vi "rszvl_core_global.vi"() -> ()   [LabVIEW 2014] (continued)
a stopped measurement at the current position in single sweep mode. The function is useful especially for trace functions MAXHold, MINHold and AVERage if the previous results are not to be cleared with Sweep Count > 0 or Average Count > 0 on restarting the measurement (INIT:IMMediate resets the previous results on restarting the measurement).\nThe single-sweep mode is automatically switched on. Synchronization to the end of the indicated number of measurements can then be performed with the command *OPC, *OPC? or *WAI. In the continuous-sweep mode, synchronization to the sweep end is not possible since the overall measurement never ends.", "Flags"={"OPC Wait"=FALSE, "Dont check status"=FALSE, "*WAI"=FALSE}, "Check Status Callback"=""}, {"Level"=3, "Descriptive Name"="Abort", "Class Only"=FALSE, "Data Type"=4, "Access"=1, "Identifier"="RSZVL_ATTR_MEAS_ABORT", "Range Table"="", "Command"="ABOR", "Read Callback"="", "Write Callback"="", "Range Callback"="", "Check Callback"="", "Rngtable Callback"="", "Coerce Callback"="", "User Callback"="", "Supported Models"="", "Instrument Options"="", "Repeated Capabilities"="", "Restricted Repeated Capabilities"="", "Help"="This attribute aborts a current measurement and resets the trigger system.\n\nAvailable Repeated Capabilities:\nNone\n\nRemote-control command(s):\nABORt", "Flags"={"OPC Wait"=FALSE, "Dont check status"=FALSE, "*WAI"=FALSE}, "Check Status Callback"=""}, {"Level"=3, "Descriptive Name"="Initiate", "Class Only"=FALSE, "Data Type"=4, "Access"=1, "Identifier"="RSZVL_ATTR_INIT", "Range Table"="", "Command"="INIT;*WAI", "Read Callback"="", "Write Callback"="", "Range Callback"="", "Check Callback"="", "Rngtable Callback"="", "Coerce Callback"="", "User Callback"="", "Supported Models"="", "Instrument Options"="", "Repeated Capabilities"="", "Restricted Repeated Capabilities"="", "Help"="This attribute initiates a new sweep.\nIn single sweep mode, synchronization to the end of the indicated number of measurements is achieved with the command *OPC. In continuous-sweep mode, synchronization to the sweep end is not possible since the overall measurement never ends.\n\nAvailable Repeated Capabilities:\nNone\n\nRemote-control command(s):\nINITiate[:IMMediate]", "Flags"={"OPC Wait"=TRUE, "Dont check status"=FALSE, "*WAI"=FALSE}, "Check Status Callback"=""}, {"Level"=3, "Descriptive Name"="Initiate Continuous", "Class Only"=FALSE, "Data Type"=3, "Access"=2, "Identifier"="RSZVL_ATTR_INIT_CONT", "Range Table"="", "Command"="INIT:CONT", "Read Callback"="", "Write Callback"="", "Range Callback"="", "Check Callback"="", "Rngtable Callback"="", "Coerce Callback"="", "User Callback"="", "Supported Models"="", "Instrument Options"="", "Repeated Capabilities"="", "Restricted Repeated Capabilities"="", "Help"="This attribute determines whether the trigger system is continuously initiated (continuous) or performs single measurements (single).\nIn the spectrum analysis mode, this setting refers to the sweep sequence (switching between continuous/single sweep).\n\nAvailable Repeated Capabilities:\nNone\n\nRemote-control command(s):\nINITiate<1|2>:CONTinuous ON | OFF", "Flags"={"OPC Wait"=FALSE, "Dont check status"=FALSE, "*WAI"=FALSE}, "Check Status Callback"=""}, {"Level"=3, "Descriptive Name"="Send Software Trigger", "Class Only"=FALSE, "Data Type"=4, "Access"=1, "Identifier"="RSZVL_ATTR_INIT_SW_TRIGGER", "Range Table"="", "Command"="*TRG", "Read Callback"="", "Write Callback"="", "Range Callback"="", "Check Callback"="", "Rngtable Callback"="", "Coerce Callback"="", "User Callback"="", "Supported Models"="", "Instrument Options"="", "Repeated Capabilities"="", "Restricted Repeated Capabilities"="", "Help"="This attribute sends a software trigger to the instrument.\n\nAvailable Repeated Capabilities:\nNone\n\nRemote-control command(s):\n*TRG", "Flags"={"OPC Wait"=TRUE, "Dont check status"=FALSE, "*WAI"=FALSE}, "Check Status Callback"=""}, {"Level"=3, "Descriptive Name"="Continue Measurement", "Class Only"=FALSE, "Data Type"=4, "Access"=1, "Identifier"="RSZVL_ATTR_INIT_CONMEAS", "Range Table"="", "Command"="INIT:CONM;*WAI", "Read Callback"="", "Write Callback"="", "Range Callback"="", "Check Callback"="", "Rngtable Callback"="", "Coerce Callback"="", "User Callback"="", "Supported Models"="", "Instrument Options"="", "Repeated Capabilities"="", "Restricted Repeated Capabilities"="", "Help"="This attribute continues a stopped measurement at the current position in single sweep mode. The function is useful especially for trace functions MAXHold, MINHold and AVERage if the previous results are not to be cleared with Sweep Count > 0 or Average Count > 0 on restarting the measurement (INIT:IMMediate resets the previous results on restarting the measurement).\nThe single-sweep mode is automatically switched on. Synchronization to the end of the indicated number of measurements can then be performed with the command *OPC, *OPC? or *WAI. In the continuous-sweep mode, synchronization to the sweep end is not possible since the overall measurement never ends.\n\nAvailable Repeated Capabilities:\nNone\n\nRemote-control command(s):\nINITiate<1|2>:CONMeas", "Flags"={"OPC Wait"=TRUE, "Dont check status"=FALSE, "*WAI"=FALSE}, "Check Status Callback"=""}, {"Level"=2, "Descriptive Name"="Average", "Class Only"=TRUE, "Data Type"=0, "Access"=0, "Identifier"="", "Range Table"="", "Command"="", "Read Callback"="", "Write Callback"="", "Range Callback"="", "Check Callback"="", "Rngtable Callback"="", "Coerce Callback"="", "User Callback"="", "Supported Models"="", "Instrument Options"="", "Repeated Capabilities"="", "Restricted Repeated Capabilities"="", "Help"="This subsystem calculates the average of the acquired data.\n\n(1) Averaging State:\nThis attribute switches on or off the average calculation for the selected trace.\n\n(2) Averaging Type:\nThis attribute selects the type of average function. If Video is selected, the logarithmic power is averaged and, if Linear is selected, the power values are averaged before they are converted to logarithmic values. The type of average calculation is equally set for all traces\n\n(3) Averaging Count:\nThis attribute defines the number of measurements which contribute to the average value.\nIt should be noted that continuous averaging will be performed after the indicated number has been reached in continuous sweep mode.\nIn single sweep mode, the sweep is stopped as soon as the indicated number of measurements (sweeps) is reached. Synchronization to the end of the indicated number of measurements is only possible in single sweep mode.\n\n(4) Averaging Count Auto:\nThis attribute is implemented only for reasons of compatibility with the FSP family. It selects a suitable number of counts for the selected measurement type.", "Flags"={"OPC Wait"=FALSE, "Dont check status"=FALSE, "*WAI"=FALSE}, "Check Status Callback"=""}, {"Level"=3, "Descriptive Name"="Averaging State", "Class Only"=FALSE, "Data Type"=3, "Access"=2, "Identifier"="RSZVL_ATTR_AVG_STATE", "Range Table"="", "Command"="SENS:AVER:STAT{Trace}", "Read Callback"="", "Write Callback"="", "Range Callback"="", "Check Callback"="", "Rngtable Callback"="", "Coerce Callback"="", "User Callback"="", "Supported Models"="", "Instrument Options"="", "Repeated Capabilities"="", "Restricted Repeated Capabilities"="", "Help"="This attribute switches on or off the average calculation for the selected trace.\n\nAvailable Repeated Capabilities:\nTrace: TR1,TR2,TR3,TR4,TR5,TR6,TR7,TR8,TR9,TR10,TR11,TR12,TR13,TR14,TR15,TR16,TR17,TR18,TR19,TR20\r\n\nRemote-control command(s):\n[SENSe<1|2>:]AVERage[:STATe<1 to 3>] ON | OFF", "Flags"={"OPC Wait"=FALSE, "Dont check status"=FALSE, "*WAI"=FALSE}, "Check Status Callback"=""}, {"Level"=3, "Descriptive Name"="Averaging Type", "Class Only"=FALSE, "Data Type"=0, "Access"=2, "Identifier"="RSZVL_ATTR_AVG_TYPE", "Range Table"="rszvl_rngAvgType", "Command"="SENS:AVER:TYPE", "Read Callback"="", "Write Callback"="", "Range Callback"="", "Check Callback"="", "Rngtable Callback"="", "Coerce Callback"="", "User Callback"="", "Supported Models"="", "Instrument Options"="", "Repeated Capabilities"="", "Restricted Repeated Capabilities"="", "Help"="This attribute selects the type of average function. If Video is selected, the logarithmic power is averaged and, if Linear is selected, the power values are averaged before they are converted to logarithmic values. The type of average calculation is equally set for all traces\n\nAvailable Repeated Capabilities:\nNone\n\nRemote-control command(s):\n[SENSe<1|2>:]AVERage:TYPE VIDeo | LINear", "Flags"={"OPC Wait"=FALSE, "Dont check status"=FALSE, "*WAI"=FALSE}, "Check Status Callback"=""}, {"Level"=3, "Descriptive Name"="Averaging Count", "Class Only"=FALSE, "Data Type"=0, "Access"=2, "Identifier"="RSZVL_ATTR_AVG_COUNT", "Range Table"="rszvl_rngAvgCount", "Command"="SENS:AVER:COUN", "Read Callback"="", "Write Callback"="", "Range Callback"="", "Check Callback"="", "Rngtable Callback"="", "Coerce Callback"="", "User Callback"="", "Supported Models"="", "Instrument Options"="", "Repeated Capabilities"="", "Restricted Repeated Capabilities"="", "Help"="This attribute defines the number of measurements which contribute to the average value.\nIt should be noted that continuous averaging will be performed after the indicated number has been reached in continuous sweep mode.\nIn single sweep mode, the sweep is stopped as soon as the indicated number of measurements (sweeps) is reached. Synchronization to the end of the indicated number of measurements is only possible in single sweep mode.\n\nAvailable Repeated Capabilities:\nNone\n\nRemote-control command(s):\n[SENSe<1|2>:]AVERage:COUNt", "Flags"={"OPC Wait"=FALSE, "Dont check status"=FALSE, "*WAI"=FALSE}, "Check Status Callback"=""}, {"Level"=3, "Descriptive Name"="Averaging Count Auto", "Class Only"=FALSE, "Data Type"=3, "Access"=2, "Identifier"="RSZVL_ATTR_AVG_COUNT_AUTO", "Range Table"="", "Command"="SENS:AVER:COUN:AUTO", "Read Callback"="", "Write Callback"="", "Range Callback"="", "Check Callback"="", "Rngtable Callback"="", "Coerce Callback"="", "User Callback"="", "Supported Models"="", "Instrument Options"="", "Repeated Capabilities"="", "Restricted Repeated Capabilities"="", "Help"="This attribute is implemented only for reasons of compatibility with the FSP family. It selects a suitable number of counts for the selected measurement type.\n\nAvailable Repeated Capabilities:\nNone\n\nRemote-control command(s):\n[SENSe<1|2>:]AVERage:COUNt:AUTO", "Flags"={"OPC Wait"=FALSE, "Dont check status"=FALSE, "*WAI"=FALSE}, "Check Status Callback"=""}, {"Level"=2, "Descriptive Name"="Bandwidth", "Class Only"=TRUE, "Data Type"=0, "Access"=0, "Identifier"="", "Range Table"="", "Command"="", "Read Callback"="", "Write Callback"="", "Range Callback"="", "Check Callback"="", "Rngtable Callback"="", "Coerce Callback"="", "User Callback"="", "Supported Models"="", "Instrument Options"="", "Repeated Capabilities"="", "Restricted Repeated Capabilities"="", "Help"="This class contains attributes configuring resolution and video bandwidth.\n\n(1) Resolution Bandwidth Filter Type:\nThis attribute sets the filter type for the resolution bandwidth.\n\n(2) Video Bandwidth Filter Type:\nThis attribute selects the position of the video filter in the signal path, provided that the resolution bandwidth is <=100 kHz:", "Flags"={"OPC Wait"=FALSE, "Dont check status"=FALSE, "*WAI"=FALSE}, "Check Status Callback"=""}, {"Level"=3, "Descriptive Name"="Resolution Bandwidth Filter Type", "Class Only"=FALSE, "Data Type"=0, "Access"=2, "Identifier"="RSZVL_ATTR_RESOLUTION_BANDWIDTH_FILTER_TYPE", "Range Table"="rszvl_rngBandFiltType", "Command"="SENS:BAND:TYPE", "Read Callback"="", "Write Callback"="", "Range Callback"="", "Check Callback"="", "Rngtable Callback"="", "Coerce Callback"="", "User Callback"="", "Supported Models"="", "Instrument Options"="", "Repeated Capabilities"="", "Restricted Repeated Capabilities"="", "Help"="This attribute sets the filter type for the resolution bandwidth.\n\nThe possible combinations of filter type and filter bandwidth are listed in Operating Manual in the table List of available channel filters in chapter 4, section Setting Bandwidths and Sweep Time- Key BW.\n\nAvailable Repeated Capabilities:\nNone\n\nRemote-control command(s):\n[SENSe<1|2>:]BANDwidth|BWIDth[:RESolution]:TYPE NORMal | FFT | CFILter | RRC | PULSe", "Flags"={"OPC Wait"=FALSE, "Dont check status"=FALSE, "*WAI"=FALSE}, "Check Status Callback"=""}, {"Level"=3, "Descriptive Name"="Video Bandwidth Filter Type", "Class Only"=FALSE, "Data Type"=0, "Access"=2, "Identifier"="RSZVL_ATTR_VIDEO_BANDWIDTH_TYPE", "Range Table"="rszvl_rngLinLog", "Command"="SENS:BAND:VID:TYPE", "Read Callback"="", "Write Callback"="", "Range Callback"="", "Check Callback"="", "Rngtable Callback"="", "Coerce Callback"="", "User Callback"="", "Supported Models"="", "Instrument Options"="", "Repeated Capabilities"="", "Restricted Repeated Capabilities"="", "Help"="This attribute selects the position of the video filter in the signal path, provided that the resolution bandwidth is <=100 kHz:\n\nAvailable Repeated Capabilities:\nNone\n\nRemote-control command(s):\n[SENSe<1|2>:]BANDwidth|BWIDth:VIDeo:TYPE LINear | LOGarithmic", "Flags"={"OPC Wait"=FALSE, "Dont check status"=FALSE, "*WAI"=FALSE}, "Check Status Callback"=""}, {"Level"=2, "Descriptive Name"="Trace", "Class Only"=TRUE, "Data Type"=0, "Access"=0, "Identifier"="", "Range Table"="", "Command"="", "Read Callback"="", "Write Callback"="", "Range Callback"="", "Check Callback"="", "Rngtable Callback"="", "Coerce Callback"="", "User Callback"="", "Supported Models"="", "Instrument Options"="", "Repeated Capabilities"="", "Restricted Repeated Capabilities"="", "Help"="Trace settings and configuration.\n\n(1) Trace State:\nThis attribute switches on or off the display of the corresponding trace.\n\n(2) Trace Reset Behavior:\nThis attribute specifies whether or not the traces with peak or minimum value detection are reset after specific parameter changes.\n\n(3) Trace Type:\nThis attribute defines the type of display and the evaluation of the traces. WRITE corresponds to the Clr/Write mode of manual operation. The trace is switched off (= BLANK in manual operation) with DISP:WIND:TRAC:STAT OFF.\n\n(4) Trace Math State:\nThis attribute switches the mathematical relation of traces on or off.\n\n(5) Trace Math Position:\nThis attribute defines the position of the result of the trace mathematics. The indication is in % of the screen height, with 100% corresponding to the upper diagram border.\n\n(6) Detector Type:\nSpecifies the detection method used to capture and process the signal. This governs the data acquisition for a particular sweep, but does not have any control over how multiple sweeps are processed.\n\n(7) Detector Type Auto:\nEnables the auto detector.", "Flags"={"OPC Wait"=FALSE, "Dont check status"=FALSE, "*WAI"=FALSE}, "Check Status Callback"=""}, {"Level"=3, "Descriptive Name"="Trace State", "Class Only"=FALSE, "Data Type"=3, "Access"=2, "Identifier"="RSZVL_ATTR_TRACE_STATE", "Range Table"="", "Command"="DISP:WIND:TRACE{Trace}", "Read Callback"="", "Write Callback"="", "Range Callback"="", "Check Callback"="", "Rngtable Callback"="", "Coerce Callback"="", "User Callback"="", "Supported Models"="", "Instrument Options"="", "Repeated Capabilities"="", "Restricted Repeated Capabilities"="", "Help"="This attribute switches on or off the display of the corresponding trace.\n\nAvailable Repeated Capabilities:\nTrace: TR1,TR2,TR3,TR4,TR5,TR6,TR7,TR8,TR9,TR10,TR11,TR12,TR13,TR14,TR15,TR16,TR17,TR18,TR19,TR20\r\n\nRemote-control command(s):\nDISPlay[:WINDow<1|2>]:TRACE<1 to 6>[:STATe]", "Flags"={"OPC Wait"=FALSE, "Dont check status"=FALSE, "*WAI"=FALSE}, "Check Status Callback"=""}, {"Level"=3, "Descriptive Name"="Trace Reset Behavior", "Class Only"=FALSE, "Data Type"=3, "Access"=2, "Identifier"="RSZVL_ATTR_TRACE_RESET_BEHAVIOR", "Range Table"="", "Command"="DISP:WIND:TRAC{Trace}:MODE:HCON", "Read Callback"="", "Write Callback"="", "Range Callback"="", "Check Callback"="", "Rngtable Callback"="", "Coerce Callback"="", "User Callback"="", "Supported Models"="", "Instrument Options"="", "Repeated Capabilities"="", "Restricted Repeated Capabilities"="", "Help"="This attribute specifies whether or not the traces with peak or minimum value detection are reset after specific parameter changes.\nUsually the measurement must be restarted after a parameter change, before an evaluation of the measurement results is performed (e.g. with a marker). In cases in which a change causes a compulsory new measurement, the trace is automatically reset in order to prevent erroneous measurements of previous measurement results (e.g. when the span changes). For applications in which this behavior is not desired, this mechanism can be switched off.\n\nAvailable Repeated Capabilities:\nTrace: TR1,TR2,TR3,TR4,TR5,TR6,TR7,TR8,TR9,TR10,TR11,TR12,TR13,TR14,TR15,TR16,TR17,TR18,TR19,TR20\r\n\nRemote-control command(s):\nDISPlay[:WINDow<1|2>]:TRACe<1 to 6>:MODE:HCONtinuous ON | OFF", "Flags"={"OPC Wait"=FALSE, "Dont check status"=FALSE, "*WAI"=FALSE}, "Check Status Callback"=""}, {"Level"=3, "Descriptive Name"="Trace Type", "Class Only"=FALSE, "Data Type"=0, "Access"=2, "Identifier"="RSZVL_ATTR_TRACE_TYPE", "Range Table"="rszvl_rngTraceMode", "Command"="DISP:WIND:TRAC{Trace}:MODe", "Read Callback"="", "Write Callback"="", "Range Callback"="", "Check Callback"="", "Rngtable Callback"="", "Coerce Callback"="", "User Callback"="", "Supported Models"="", "Instrument Options"="", "Repeated Capabilities"="", "Restricted Repeated Capabilities"="", "Help"="This attribute defines the type of display and the evaluation of the traces. WRITE corresponds to the Clr/Write mode of manual operation. The trace is switched off (= BLANK in manual operation) with DISP:WIND:TRAC:STAT OFF.\nThe number of measurements for AVERage, MAXHold and MINHold is defined with the command SENSe:AVERage:COUNt or SENSe:SWEep:COUNt. It should be noted that synchronization to the end of the indicated number of measurements is only possible in single sweep mode. If calculation of average values is active, selection between logarithmic and linear averaging is possible. For more detail see command SENSe:AVERage:TYPE.\n\nAvailable Repeated Capabilities:\nTrace: TR1,TR2,TR3,TR4,TR5,TR6,TR7,TR8,TR9,TR10,TR11,TR12,TR13,TR14,TR15,TR16,TR17,TR18,TR19,TR20\r\n\nRemote-control command(s):\nDISPlay[:WINDow<1|2>]:TRACe<1 to 6>:MODE WRITe | VIEW | AVERage | MAXHold | MINHold | BLANk", "Flags"={"OPC Wait"=FALSE, "Dont check status"=FALSE, "*WAI"=FALSE}, "Check Status Callback"=""}, {"Level"=3, "Descriptive Name"="Trace Math State", "Class Only"=FALSE, "Data Type"=3, "Access"=2, "Identifier"="RSZVL_ATTR_TRACE_MATH_STATE", "Range Table"="", "Command"="CALC:MATH:STAT", "Read Callback"="", "Write Callback"="", "Range Callback"="", "Check Callback"="", "Rngtable Callback"="", "Coerce Callback"="", "User Callback"="", "Supported Models"="", "Instrument Options"="", "Repeated Capabilities"="", "Restricted Repeated Capabilities"="", "Help"="This attribute switches the mathematical relation of traces on or off.\n\nAvailable Repeated Capabilities:\nNone\n\nRemote-control command(s):\nCALCulate<1|2>:MATH:STATe ON | OFF", "Flags"={"OPC Wait"=FALSE, "Dont check status"=FALSE, "*WAI"=FALSE}, "Check Status Callback"=""}, {"Level"=3, "Descriptive Name"="Trace Math Position", "Class Only"=FALSE, "Data Type"=1, "Access"=2, "Identifier"="RSZVL_ATTR_TRACE_MATH_POSITION", "Range Table"="rszvl_rngTraceMathPosition", "Command"="CALC:MATH:POS", "Read Callback"="", "Write Callback"="", "Range Callback"="", "Check Callback"="", "Rngtable Callback"="", "Coerce Callback"="", "User Callback"="", "Supported Models"="", "Instrument Options"="", "Repeated Capabilities"="", "Restricted Repeated Capabilities"="", "Help"="This attribute defines the position of the result of the trace mathematics. The indication is in % of the screen height, with 100% corresponding to the upper diagram border.\n\nAvailable Repeated Capabilities:\nNone\n\nRemote-control command(s):\nCALCulate<1|2>:MATH:POSition", "Flags"={"OPC Wait"=FALSE, "Dont check status"=FALSE, "*WAI"=FALSE}, "Check Status Callback"=""}, {"Level"=3, "Descriptive Name"="Detector Type", "Class Only"=FALSE, "Data Type"=0, "Access"=2, "Identifier"="RSZVL_ATTR_DETECTOR_TYPE", "Range Table"="rszvl_rngDetectorTypeRangeTable", "Command"="SENS:DET{Trace}:FUNC", "Read Callback"="", "Write Callback"="", "Range Callback"="", "Check Callback"="", "Rngtable Callback"="", "Coerce Callback"="", "User Callback"="", "Supported Models"="", "Instrument Options"="", "Repeated Capabilities"="", "Restricted Repeated Capabilities"="", "Help"="Specifies the detection method used to capture and process the signal. This governs the data acquisition for a particular sweep, but does not have any control over how multiple sweeps are processed.\n\nAvailable Repeated Capabilities:\nTrace: TR1,TR2,TR3,TR4,TR5,TR6,TR7,TR8,TR9,TR10,TR11,TR12,TR13,TR14,TR15,TR16,TR17,TR18,TR19,TR20\r\n\nRemote-control command(s):\n[SENSe<1|2>:]DETector<1 to 6>[:FUNCtion] APEak | NEGative | POSitive | SAMPle | RMS |", "Flags"={"OPC Wait"=FALSE, "Dont check status"=FALSE, "*WAI"=FALSE}, "Check Status Callback"=""}, {"Level"=3, "Descriptive Name"="Detector Type Auto", "Class Only"=FALSE, "Data Type"=3, "Access"=2, "Identifier"="RSZVL_ATTR_DETECTOR_TYPE_AUTO", "Range Table"="", "Command"="SENS:DET{Trace}:AUTO", "Read Callback"="", "Write Callback"="", "Range Callback"="", "Check Callback"="", "Rngtable Callback"="", "Coerce Callback"="", "User Callback"="", "Supported Models"="", "Instrument Options"="", "Repeated Capabilities"="", "Restricted Repeated Capabilities"="", "Help"="Enables the auto detector.\nNote:\nWhen the RSZVL_ATTR_DETECTOR_TYPE_AUTO attribute is set to True, the relationship between the RSZVL_ATTR_TRACE_TYPE attribute and the RSZVL_ATTR_DETECTOR_TYPE attribute is not defined.\n\nAvailable Repeated Capabilities:\nTrace: TR1,TR2,TR3,TR4,TR5,TR6,TR7,TR8,TR9,TR10,TR11,TR12,TR13,TR14,TR15,TR16,TR17,TR18,TR19,TR20\r\n\nRemote-control command(s):\n[SENSe<1|2>:]DETector<1 to 6>[:FUNCtion]:AUTO ON | OFF", "Flags"={"OPC Wait"=FALSE, "Dont check status"=FALSE, "*WAI"=FALSE}, "Check Status Callback"=""}, {"Level"=2, "Descriptive Name"="Calibration", "Class Only"=TRUE, "Data Type"=0, "Access"=0, "Identifier"="", "Range Table"="", "Command"="", "Read Callback"="", "Write Callback"="", "Range Callback"="", "Check Callback"="", "Rngtable Callback"="", "Coerce Callback"="", "User Callback"="", "Supported Models"="", "Instrument Options"="", "Repeated Capabilities"="", "Restricted Repeated Capabilities"="", "Help"="(1) Calibration:\nThis attribute initiates the acquisition of system error correction data. A 0 is returned if the acquisition was successful.\n\n(2) Calibration Abort:\nThis atribute aborts the acquisition of correction data and restores the last complete correction data set.\n\n(3) Calibration Result Query:\nThis attribute outputs the results of the correction data acquisition.\n\n(4) Calibration State:\nThis attribute determines whether the current calibration data are taken into account by the instrument (ON) or not (OFF).", "Flags"={"OPC Wait"=FALSE, "Dont check status"=FALSE, "*WAI"=FALSE}, "Check Status Callback"=""}, {"Level"=3, "Descriptive Name"="Calibration Check", "Class Only"=FALSE, "Data Type"=0, "Access"=0, "Identifier"="RSZVL_ATTR_CALIBRATION_CHECK", "Range Table"="rszvl_rngCalibration", "Command"="*CLS;CAL?", "Read Callback"="", "Write Callback"="", "Range Callback"="", "Check Callback"="", "Rngtable Callback"="", "Coerce Callback"="", "User Callback"="", "Supported Models"="", "Instrument Options"="", "Repeated Capabilities"="", "Restricted Repeated Capabilities"="", "Help"="This attribute initiates the acquisition of system error correction data. A 0 is returned if the acquisition was successful.\n\nNote: During the acquisition of correction data the instrument does not accept any remote control commands, except\n*RST\nCALibration:ABORt\n\nAvailable Repeated Capabilities:\nNone\n\nRemote-control command(s):\nCALibration[:ALL]?", "Flags"={"OPC Wait"=FALSE, "Dont check status"=TRUE, "*WAI"=FALSE}, "Check Status Callback"=""}, {"Level"=3, "Descriptive Name"="Calibration Start", "Class Only"=FALSE, "Data Type"=4, "Access"=1, "Identifier"="RSZVL_ATTR_CALIBRATION", "Range Table"="", "Command"="*CLS;CAL ALL", "Read Callback"="", "Write Callback"="", "Range Callback"="", "Check Callback"="", "Rngtable Callback"="", "Coerce Callback"="", "User Callback"="", "Supported Models"="", "Instrument Options"="", "Repeated Capabilities"="", "Restricted Repeated Capabilities"="", "Help"="This attribute initiates the acquisition of system error correction data. \n\nNote: Attribute doesn't wait to completation. This selection allows to use Calibration Abort if necessary. Use viReadSTB to check Operation complete.\n\nAvailable Repeated Capabilities:\nNone\n\nRemote-control command(s):\nCALibration[:ALL]", "Flags"={"OPC Wait"=FALSE, "Dont check status"=TRUE, "*WAI"=FALSE}, "Check Status Callback"=""}, {"Level"=3, "Descriptive Name"="Calibration Abort", "Class Only"=FALSE, "Data Type"=4, "Access"=1, "Identifier"="RSZVL_ATTR_CALIBRATION_ABORT", "Range Table"="", "Command"="CAL:ABOR", "Read Callback"="", "Write Callback"="", "Range Callback"="", "Check Callback"="", "Rngtable Callback"="", "Coerce Callback"="", "User Callback"="", "Supported Models"="", "Instrument Options"="", "Repeated Capabilities"="", "Restricted Repeated Capabilities"="", "Help"="This atribute aborts the acquisition of correction data and restores the last complete correction data set.\n\nAvailable Repeated Capabilities:\nNone\n\nRemote-control command(s):\nCALibration:ABORt", "Flags"={"OPC Wait"=TRUE, "Dont check status"=FALSE, "*WAI"=FALSE}, "Check Status Callback"=""}, {"Level"=3, "Descriptive Name"="Calibration Result Query", "Class Only"=FALSE, "Data Type"=2, "Access"=0, "Identifier"="RSZVL_ATTR_CALIBRATION_RESULT_QUERY", "Range Table"="", "Command"="CAL:RES?", "Read Callback"="", "Write Callback"="", "Range Callback"="", "Check Callback"="", "Rngtable Callback"="", "Coerce Callback"="", "User Callback"="", "Supported Models"="", "Instrument Options"="", "Repeated Capabilities"="", "Restricted Repeated Capabilities"="", "Help"="This attribute outputs the results of the correction data acquisition. The lines of the result table (see section Recording the correction data of FSQ - CAL key) are output as string data separated by\ncommas:\nTotal Calibration Status: PASSED,Date (dd/mm/yyyy): 12/07/1999, Time: 16:24:54,Runtime:00.06\n\nAvailable Repeated Capabilities:\nNone\n\nRemote-control command(s):\nCALibration:RESult?", "Flags"={"OPC Wait"=FALSE, "Dont check status"=FALSE, "*WAI"=FALSE}, "Check Status Callback"=""}, {"Level"=3, "Descriptive Name"="Calibration State", "Class Only"=FALSE, "Data Type"=3, "Access"=2, "Identifier"="RSZVL_ATTR_CALIBRATION_STATE", "Range Table"="", "Command"="CAL:STAT", "Read Callback"="", "Write Callback"="", "Range Callback"="", "Check Callback"="", "Rngtable Callback"="", "Coerce Callback"="", "User Callback"="", "Supported Models"="", "Instrument Options"="", "Repeated Capabilities"="", "Restricted Repeated Capabilities"="", "Help"="This attribute determines whether the current calibration data are taken into account by the instrument (ON) or not (OFF).\n\nAvailable Repeated Capabilities:\nNone\n\nRemote-control command(s):\nCALibration:STATe ON | OFF", "Flags"={"OPC Wait"=FALSE, "Dont check status"=FALSE, "*WAI"=FALSE}, "Check Status Callback"=""}, {"Level"=2, "Descriptive Name"="User Port", "Class Only"=TRUE, "Data Type"=0, "Access"=0, "Identifier"="", "Range Table"="", "Command"="", "Read Callback"="", "Write Callback"="", "Range Callback"="", "Check Callback"="", "Rngtable Callback"="", "Coerce Callback"="", "User Callback"="", "Supported Models"="", "Instrument Options"="", "Repeated Capabilities"="", "Restricted Repeated Capabilities"="", "Help"="(1) User Ports State:\nThis attribute toggles the control lines of the user ports between INPut and OUTPut. With ON, the user port is switched to INPut, with OFF to OUTPut.\n\n(2) User Ports Control Lines:\nThis attribute queries the control lines of the user ports.\n\n(3) User Ports Output Control Lines:\nThis attribute sets the control lines of the user ports. The user port is written to with the given binary pattern. If the user port is programmed to INPut instead of OUTPut, the output value is temporarily stored.", "Flags"={"OPC Wait"=FALSE, "Dont check status"=FALSE, "*WAI"=FALSE}, "Check Status Callback"=""}, {"Level"=3, "Descriptive Name"="User Ports State", "Class Only"=FALSE, "Data Type"=3, "Access"=2, "Identifier"="RSZVL_ATTR_INP_UPORT_STATE", "Range Table"="", "Command"="INP:UPOR:STAT", "Read Callback"="", "Write Callback"="", "Range Callback"="", "Check Callback"="", "Rngtable Callback"="", "Coerce Callback"="", "User Callback"="", "Supported Models"="", "Instrument Options"="", "Repeated Capabilities"="", "Restricted Repeated Capabilities"="", "Help"="This attribute toggles the control lines of the user ports between INPut and OUTPut. With ON, the user port is switched to INPut, with OFF to OUTPut.\n\nAvailable Repeated Capabilities:\nNone\n\nRemote-control command(s):\nINPut<1|2>:UPORt:STATe", "Flags"={"OPC Wait"=FALSE, "Dont check status"=FALSE, "*WAI"=FALSE}, "Check Status Callback"=""}, {"Level"=3, "Descriptive Name"="User Ports Control Lines", "Class Only"=FALSE, "Data Type"=2, "Access"=0, "Identifier"="RSZVL_ATTR_INP_UPORT_VALUE", "Range Table"="", "Command"="INP:UPOR?", "Read Callback"="rszvl_stringToBin_ReadCallback.vi", "Write Callback"="", "Range Callback"="", "Check Callback"="", "Rngtable Callback"="", "Coerce Callback"="", "User Callback"="", "Supported Models"="", "Instrument Options"="", "Repeated Capabilities"="", "Restricted Repeated Capabilities"="", "Help"="This attribute queries the control lines of the user ports.\n\nAvailable Repeated Capabilities:\nNone\n\nRemote-control command(s):\nINPut<1|2>:UPORt[:VALue]?", "Flags"={"OPC Wait"=FALSE, "Dont check status"=FALSE, "*WAI"=FALSE}, "Check Status Callback"=""}, {"Level"=3, "Descriptive Name"="User Ports Output Control Lines", "Class Only"=FALSE, "Data Type"=2, "Access"=2, "Identifier"="RSZVL_ATTR_OUT_UPORT_VALUE", "Range Table"="", "Command"="OUTP:UPOR", "Read Callback"="rszvl_stringToBin_ReadCallback.vi", "Write Callback"="rszvl_stringToBin_WriteCallback.vi", "Range Callback"="", "Check Callback"="", "Rngtable Callback"="", "Coerce Callback"="", "User Callback"="", "Supported Models"="", "Instrument Options"="", "Repeated Capabilities"="", "Restricted Repeated Capabilities"="", "Help"="This attribute sets the control lines of the user ports. The user port is written to with the given binary pattern. If the user port is programmed to INPut instead of OUTPut, the output value is temporarily stored.\n\nAvailable Repeated Capabilities:\nNone\n\nRemote-control command(s):\nOUTPut:UPORt[:VALue]", "Flags"={"OPC Wait"=FALSE, "Dont check status"=FALSE, "*WAI"=FALSE}, "Check Status Callback"=""}, {"Level"=1, "Descriptive Name"="Display Control", "Class Only"=TRUE, "Data Type"=0, "Access"=0, "Identifier"="", "Range Table"="", "Command"="", "Read Callback"="", "Write Callback"="", "Range Callback"="", "Check Callback"="", "Rngtable Callback"="", "Coerce Callback"="", "User Callback"="", "Supported Models"="", "Instrument Options"="", "Repeated Capabilities"="", "Restricted Repeated Capabilities"="", "Help"="(1) Display Reference Value:\nIf the external generator control option is mounted and the normalization in the NETWORK mode is activated, this value defines the power value assigned to the reference position. This value corresponds to the parameter REFERENCE VALUE in manual operation. The numeric suffix is irrelevant.\n\n(2) Display Reference Position:\nThis attribute defines the position of the reference value. The numeric suffix is irrelevant.\n\n(3) Display Frequency State:\nThis attribute switches the X axis annotation on or off.\n\n(4) Display Time State:\nThis attribute switches on or off the screen display of date and time.\n\n(5) Display Power Save State:\nThis attribute switches on or off the power-save mode of the display. With the power-save mode activated the display including backlight is completely switched off after the elapse of the response time (see command DISPlay:PSAVe:HOLDoff).\n\nNote: This mode is recommended for preserving the display especially if the instrument is exclusively operated via remote control.\n\n(6) Display Power Save Holdoff:\nThis attribute sets the holdoff time for the power-save mode of the display. The available value range is 1 to 60 minutes, the resolution 1 minute. The entry is dimensionless.\n\n(7) Display Window Size:\nThis attribute switches the measurement window for channel and adjacent-channel power measurements to full screen or half screen.\n\n(8) Display Color Preset:\nThis attribute resets the screen colors of all display items to their default settings. Two default settings DEFault1 and DEFault2 are available. The numeric suffix of CMAP is irrelevant.\n\n(9) Display Color Predefined:\nThis attribute defines the color table of the instrument using predefined color values. Each numeric suffix of CMAP is assigned one or several graphical elements which can be modified by varying the corresponding color setting.\nThe same assignment as for DISPlay:CMAP<1 to 26>:HSL applies.\n\n(10) Display Log Range:\nThis attribute defines the display range of the Y axis (level axis) with logarithmic scaling (DISP:TRAC:Y:SPAC LOG).\nFor linear scaling, (DISP:TRAC:Y:SPAC LIN | PERC) the display range is fixed and cannot be modified.\n\n(11) Display Amplitude Grid Mode:\nThis attribute defines the scale type of the Y axis (absolute or relative).\nWhen SYSTem:DISPlay is set to OFF, this command has no immediate effect on the screen. The numeric suffix is irrelevant.\n\n(12) Display During Single Sweep:\nThis attribute configures the behaviour of the display during a single sweep.\nINITiate:DISPlay OFF means that the display is switched off during the measurement, INITiate:DISPlay ON means that the display is switched on during the measurement.\n\n(13) Display Update:\nThis attribute switches on or off the update of all display elements during remote control.\n\nNote: \n(1) The best performance is obtained when the display output is switched off during remote control.\n\n(14) Configure Display Unit Power:\nThis attribute selects the unit for power.", "Flags"={"OPC Wait"=FALSE, "Dont check status"=FALSE, "*WAI"=FALSE}, "Check Status Callback"=""}, {"Level"=2, "Descriptive Name"="Display Reference Value", "Class Only"=FALSE, "Data Type"=1, "Access"=2, "Identifier"="RSZVL_ATTR_DISP_REF_VALUE", "Range Table"="", "Command"="DISP:WIND:TRAC:Y:RVAL", "Read Callback"="", "Write Callback"="", "Range Callback"="", "Check Callback"="", "Rngtable Callback"="", "Coerce Callback"="", "User Callback"="", "Supported Models"="", "Instrument Options"="", "Repeated Capabilities"="", "Restricted Repeated Capabilities"="", "Help"="If the external generator control option is mounted and the normalization in the NETWORK mode is activated, this value defines the power value assigned to the reference position. This value corresponds to the parameter REFERENCE VALUE in manual operation. The numeric suffix is irrelevant.\n\nAvailable Repeated Capabilities:\nNone\n\nRemote-control command(s):\nDISPlay[:WINDow<1|2>]:TRACE<1 to 6>:Y[:SCALe]:RVALue", "Flags"={"OPC Wait"=FALSE, "Dont check status"=FALSE, "*WAI"=FALSE}, "Check Status Callback"=""}, {"Level"=2, "Descriptive Name"="Display Reference Position", "Class Only"=FALSE, "Data Type"=1, "Access"=2, "Identifier"="RSZVL_ATTR_DISP_REF_POSITION", "Range Table"="rszvl_rngPct", "Command"="DISP:WIND:TRAC:Y:RPOS", "Read Callback"="", "Write Callback"="", "Range Callback"="", "Check Callback"="", "Rngtable Callback"="", "Coerce Callback"="", "User Callback"="", "Supported Models"="", "Instrument Options"="", "Repeated Capabilities"="", "Restricted Repeated Capabilities"="", "Help"="This attribute defines the position of the reference value. The numeric suffix is irrelevant.\n\nAvailable Repeated Capabilities:\nNone\n\nRemote-control command(s):\nDISPlay[:WINDow<1|2>]:TRACe<1 to 6>:Y[:SCALe]:RPOSition", "Flags"={"OPC Wait"=FALSE, "Dont check status"=FALSE, "*WAI"=FALSE}, "Check Status Callback"=""}, {"Level"=2, "Descriptive Name"="Display Frequency State", "Class Only"=FALSE, "Data Type"=3, "Access"=2, "Identifier"="RSZVL_ATTR_DISP_FREQ_STATE", "Range Table"="", "Command"="DISP:ANN:FREQ", "Read Callback"="", "Write Callback"="", "Range Callback"="", "Check Callback"="", "Rngtable Callback"="", "Coerce Callback"="", "User Callback"="", "Supported Models"="", "Instrument Options"="", "Repeated Capabilities"="", "Restricted Repeated Capabilities"="", "Help"="This attribute switches the X axis annotation on or off.\n\nAvailable Repeated Capabilities:\nNone\n\nRemote-control command(s):\nDISPlay:ANNotation:FREQuency ON | OFF", "Flags"={"OPC Wait"=FALSE, "Dont check status"=FALSE, "*WAI"=FALSE}, "Check Status Callback"=""}, {"Level"=2, "Descriptive Name"="Display Time State", "Class Only"=FALSE, "Data Type"=3, "Access"=2, "Identifier"="RSZVL_ATTR_DISP_TIME_STATE", "Range Table"="", "Command"="DISP:TIME", "Read Callback"="", "Write Callback"="", "Range Callback"="", "Check Callback"="", "Rngtable Callback"="", "Coerce Callback"="", "User Callback"="", "Supported Models"="", "Instrument Options"="", "Repeated Capabilities"="", "Restricted Repeated Capabilities"="", "Help"="This attribute switches on or off the screen display of date and time.\n\nAvailable Repeated Capabilities:\nNone\n\nRemote-control command(s):\nDISPlay[:WINDow<1|2>]:TIME ON | OFF", "Flags"={"OPC Wait"=FALSE, "Dont check status"=FALSE, "*WAI"=FALSE}, "Check Status Callback"=""}, {"Level"=2, "Descriptive Name"="Display Power Save State", "Class Only"=FALSE, "Data Type"=3, "Access"=2, "Identifier"="RSZVL_ATTR_DISP_PWR_SAVE_STATE", "Range Table"="", "Command"="DISP:PSAV", "Read Callback"="", "Write Callback"="", "Range Callback"="", "Check Callback"="", "Rngtable Callback"="", "Coerce Callback"="", "User Callback"="", "Supported Models"="", "Instrument Options"="", "Repeated Capabilities"="", "Restricted Repeated Capabilities"="", "Help"="This attribute switches on or off the power-save mode of the display. With the power-save mode activated the display including backlight is completely switched off after the elapse of the response time (see command DISPlay:PSAVe:HOLDoff).\n\nNote: This mode is recommended for preserving the display especially if the instrument is exclusively operated via remote control.\n\nAvailable Repeated Capabilities:\nNone\n\nRemote-control command(s):\nDISPlay:PSAVe[:STATe] ON | OFF", "Flags"={"OPC Wait"=FALSE, "Dont check status"=FALSE, "*WAI"=FALSE}, "Check Status Callback"=""}, {"Level"=2, "Descriptive Name"="Display Power Save Holdoff", "Class Only"=FALSE, "Data Type"=0, "Access"=2, "Identifier"="RSZVL_ATTR_DISP_PWR_SAVE_HOLDOFF", "Range Table"="rszvl_rngDISPConfPowSave", "Command"="DISP:PSAV:HOLD", "Read Callback"="", "Write Callback"="", "Range Callback"="", "Check Callback"="", "Rngtable Callback"="", "Coerce Callback"="", "User Callback"="", "Supported Models"="", "Instrument Options"="", "Repeated Capabilities"="", "Restricted Repeated Capabilities"="", "Help"="This attribute sets the holdoff time for the power-save mode of the display. The available value range is 1 to 60 minutes, the resolution 1 minute. The entry is dimensionless.\n\nAvailable Repeated Capabilities:\nNone\n\nRemote-control command(s):\nDISPlay:PSAVe:HOLDoff", "Flags"={"OPC Wait"=FALSE, "Dont check status"=FALSE, 
